vi "zmq_z85_decode.vi"(3 "error in":errorcluster, 5 "encoded string":string) -> (0 "error out":errorcluster, 2 "data out":u8[](array[numeric]))   [LabVIEW 2020, in "zeromq.lvlib"]
doc: "Queries and returns the version of ZeroMQ currently loaded as both a string and struct.\n\nDetailed API documentation: http://api.zeromq.org/3-2:zmq-version"
uses:
  zeromq.lvlib
panel:
  # "ØMQ"
  # "labview"
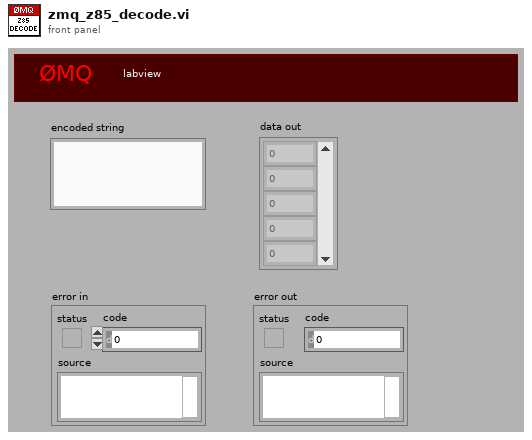
[diagram p1: front panel]
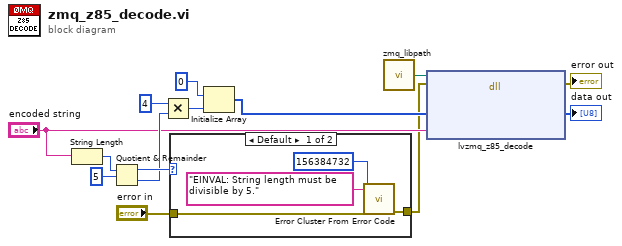
[diagram p0: block diagram]
diagram:
  n1 = String Length(string="encoded string") -> (length=w3:i32)
  n2 = Quotient & Remainder(x=w3, y=5) -> (x-y*floor(x/y)=w9:i32, floor(x/y)=w7:i32)
  n3 = Multiply(x=4, y=w7) -> (x*y=w5:i32)
  n4 = case shown="Default" w9 {
    tunnel: "error in" -> [w16 w19]
    tunnel: [w15 w19] -> w1
    frame Default {
      n5 = call "Error Cluster From Error Code.vi"("error in (no error)"=w16, "error message (\"\")"="EINVAL: String length must be divisible by 5." ("error message (\"\")"), "error code (0)"=156384732) -> ("error out"=w15:errorcluster)  [unwired: 6 in]
    }
    frame 0 {
      # "Divisible by 5, is ok"
    }
  }
  n6 = Initialize Array(u8 0 ("element"), w5) -> (w10:u8[])
  n7 = call "zmq_libpath.vi"() -> ("path"=w13:path)
  n8 = dll-call lib="?" fn="lvzmq_z85_decode" ("zmq_labview.dll:lvzmq_socket")(path in=w13, error in=w1, "dest"=w10, "src"="encoded string") -> (error out=→"error out":errorcluster, "dest"=→"data out":u8[])  [unwired: 3 in, 1 out]
